vi "Periodic Tasks.vi"(8 "error in":errorcluster) -> ()   [LabVIEW 2019]
doc: "This VI runs in parallel to other tasks. It can contain as many user-defined periodic loops as you need. These can carry out PID or other sorts of timed response."
uses:
  <vilib>/Rock Robotics/WPI/Utilities/WPI_GetSetVariantRefNum.vi
  Robot Global Data.vi
  <vilib>/Rock Robotics/Network Tables/NT Read Number.vi
  <vilib>/Rock Robotics/Network Tables/NT Write Number.vi
  <vilib>/Rock Robotics/WPI/Ultrasonic/WPI_SonarSRF04DigitalGetRange.vi
  <vilib>/Rock Robotics/WPI/Ultrasonic/WPI_SonarSRF04DigitalRefNum Registry Get.vi
panel:
  out "Distance":dbl
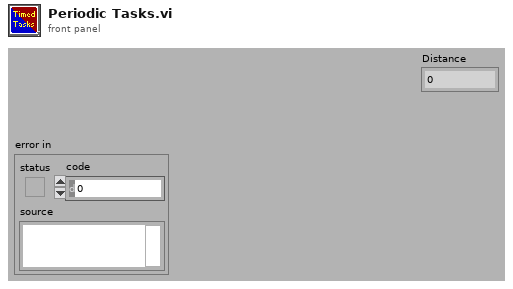
[diagram p1: front panel]
types:
  T1 = typedef "WPI_ServoDeviceRef.ctl" = cluster{"DeviceStatus":errorcluster, "PWM Channel":T2, "DeadBand":T3}
  T2 = typedef "FPGA_DIOPWMChannel.ctl" = enum8{"PWM 0", "PWM 1", "PWM 2", "PWM 3", "PWM 4", "PWM 5", "PWM 6", "PWM 7", "PWM 8", "PWM 9", "PWM MXP 0", "PWM MXP 1", "PWM MXP 2", "PWM MXP 3", "PWM MXP 4", "PWM MXP 5", "PWM MXP 6", "PWM MXP 7", "PWM MXP 8", "PWM MXP 9", "Invalid"}
  T3 = typedef "WPI_PWMDeadband.ctl" = cluster{"Name":string, "maxPositivePwm":i32, "minPositivePwm":i32, "centerPwm":i32, "maxNegativePwm":i32, "minNegativePwm":i32, "angularRange":u16}
  T4 = typedef "WPI_UltrasonicDeviceRef.ctl" = cluster{"DevStatus":errorcluster, "Ping Channel":T5, "Echo Channel":T5, "CntIndex":T6}
  T5 = typedef "FPGA_DIOChannel.ctl" = enum8{"DIO 0", "DIO 1", "DIO 2", "DIO 3", "DIO 4", "DIO 5", "DIO 6", "DIO 7", "DIO 8", "DIO 9", "DIO MXP 0", "DIO MXP 1", "DIO MXP 2", "DIO MXP 3", "DIO MXP 4", "DIO MXP 5", "DIO MXP 6", "DIO MXP 7", "DIO MXP 8", "DIO MXP 9", "DIO MXP 10", "DIO MXP 11", "DIO MXP 12", "DIO MXP 13", "DIO MXP 14", "DIO MXP 15", "SPI Port CS1", "SPI Port CS2", "SPI Port CS3", "SPI Port MISO", "SPI Port MOSI", "Invalid"}
  T6 = typedef "FPGA_CounterCtrSystemIndex.ctl" = enum8{"Ctr 0", "Ctr 1", "Ctr 2", "Ctr 3", "Ctr 4", "Ctr 5", "Ctr 6", "Ctr 7", "Invalid"}
  T7 = typedef "WPI_JoystickDevRef.ctl" = cluster{"Device":T8}
  T8 = typedef "WPI_JoystickDeviceEnum.ctl" = enum16{"USB 0", "USB 1", "USB 2", "USB 3", "USB 4", "USB 5"}
  T9 = typedef "WPI_RobotDriveDevRef.ctl" = cluster{"DevStatus":errorcluster, "Motors[]":T10[], "Square Inputs":bool, "Max Output":dbl}
  T10 = typedef "WPI_MotorControlDeviceRef.ctl" = cluster{"DeviceStatus":errorcluster, "Type":T11, "PWM":cluster{"PWM Channel":T2, "DeadBand":T3}, "CAN":cluster{"Device Number":u8, "SetOutput VI Ref":variant, "GetOutput VI Ref":variant, "Enable VI Ref":variant, "Disable VI Ref":variant, "Data":variant}, "Invert":bool, "DIO PWM":cluster{"PWM \"Enable\" Channel":T2, "DIOChannel":T5, "PWM Rate":dbl}}
  T11 = typedef "WPI_MotorControlType.ctl" = enum16{"PWM", "CAN", "DIO PWM"}
  T12 = typedef "WPI_GyroDevRef.ctl" = cluster{"DevStatus":errorcluster, "Analog Channel":T13, "Gain (VoltsPerDegree/Second)":dbl, "Gyro Type":enum16{"Analog", "XRS450"}, "Handle":i32, "SPI Bus":T14, "Device Found":bool, "Sample Rate":dbl, "Calibrate On Open":bool, "Offset":dbl}
  T13 = typedef "FPGA_AIChannel.ctl" = enum8{"AI 0", "AI 1", "AI 2", "AI 3", "AI MXP 0", "AI MXP 1", "AI MXP 2", "AI MXP 3", "Invalid"}
  T14 = typedef "spi_bus.ctl" = enum16{"SPI On-Board, CS0", "SPI On-Board, CS1", "SPI On-Board, CS2", "SPI On-Board, CS3", "SPI MXP", "Invalid"}
  T15 = cluster{"JoystickDevRef":T7, "RobotDriveDevRef":T9}
  T16 = typedef "WPI_EncoderDevRef.ctl" = cluster{"DevStatus":errorcluster, "EncoderIndex":T17, "CounterIndex":T6, "DistancePerCount":dbl, "Decoding Type":T18}
  T17 = typedef "FPGA_EncoderIdx.ctl" = enum8{"Enc 0", "Enc 1", "Enc 2", "Enc 3", "Enc 4", "Enc 5", "Enc 6", "Enc 7", "Invalid"}
  T18 = typedef "WPI_EncoderType.ctl" = enum16{"1x", "2x", "4x"}
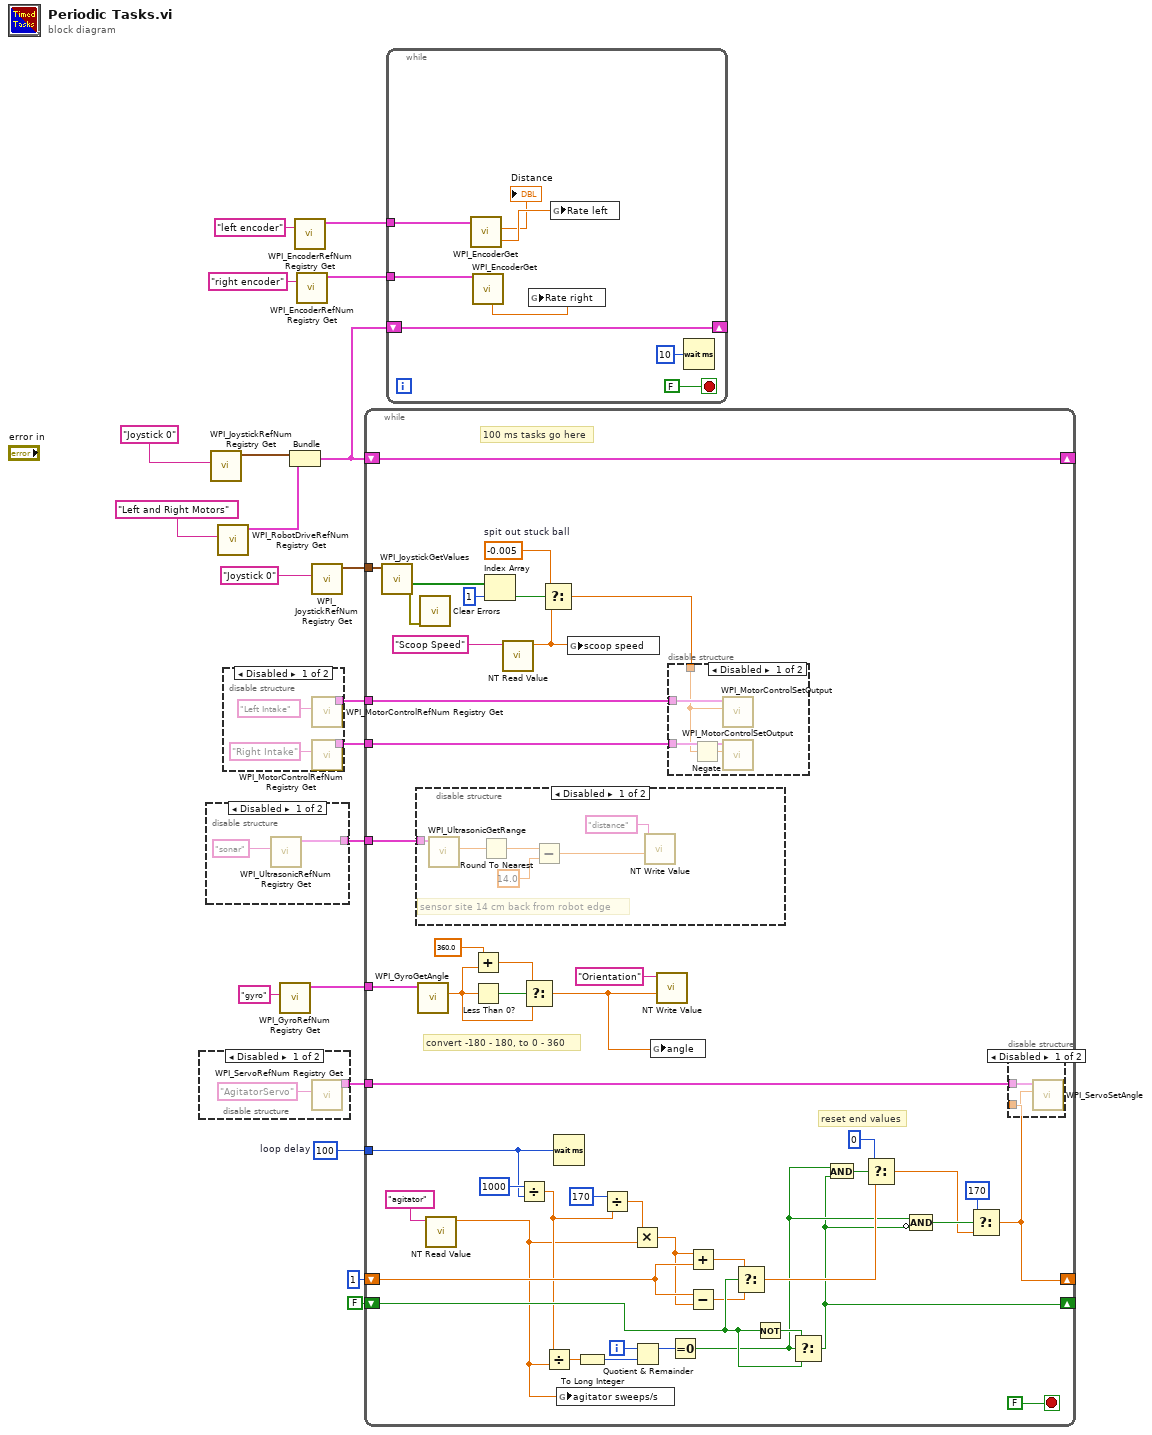
[diagram p0: block diagram]
diagram:
  w8 = u32 100  # loop delay
  n1 = disable-structure shown="Disabled" {
    disable-tunnel: [w21 _] -> w15
    frame Disabled {
      n2 = call <vilib>:"WPI_ServoRefNum Registry Get.vi"("refnum name"="AgitatorServo") -> ("ServoDeviceRef"=w21:T1)  [unwired: 9 in, 1 out]
    }
    frame Enabled {
    }
  }
  n3 = disable-structure shown="Disabled" {
    disable-tunnel: [w23 _] -> w7
    frame Disabled {
      n4 = call-poly <vilib>:"WPI_UltrasonicRefNum Registry Get.vi"("refnum name"="sonar") -> ("SonarSRF04DevRef"=w23:T4)  [unwired: 9 in, 1 out]
    }
    frame Enabled {
    }
  }
  n5 = call <vilib>:"WPI_JoystickRefNum Registry Get.vi"("refnum name"="Joystick 0") -> ("JoystickDevRef"=w18:T7)  [unwired: 1 in, 9 out]
  n6 = call <vilib>:"WPI_RobotDriveRefNum Registry Get.vi"("refnum name"="Left and Right Motors") -> ("RobotDriveDevRef"=w17:T9)  [unwired: 1 in, 9 out]
  n7 = disable-structure shown="Disabled" {
    disable-tunnel: [w28 _] -> w12
    disable-tunnel: [w25 _] -> w11
    frame Disabled {
      n8 = call <vilib>:"WPI_MotorControlRefNum Registry Get.vi"("refnum name"="Left Intake") -> ("MotorControlDevRef"=w28:T10)  [unwired: 9 in, 1 out]
      n9 = call <vilib>:"WPI_MotorControlRefNum Registry Get.vi"("refnum name"="Right Intake") -> ("MotorControlDevRef"=w25:T10)  [unwired: 9 in, 1 out]
    }
    frame Enabled {
    }
  }
  n10 = call <vilib>:"WPI_GyroRefNum Registry Get.vi"("refnum name"="gyro") -> ("GyroDevRef"=w5:T12)  [unwired: 9 in, 1 out]
  n11 = Bundle("JoystickDevRef"=w18, "RobotDriveDevRef"=w17) -> (w16:T15)  [unwired: 1 out]
  n12 = call <vilib>:"WPI_EncoderRefNum Registry Get.vi"("refnum name"="left encoder") -> ("EncoderDevRef"=w1:T16)  [unwired: 9 in, 1 out]
  n13 = call <vilib>:"WPI_EncoderRefNum Registry Get.vi"("refnum name"="right encoder") -> ("EncoderDevRef"=w4:T16)  [unwired: 9 in, 1 out]
  n14 = call <vilib>:"WPI_JoystickRefNum Registry Get.vi"("refnum name"="Joystick 0") -> ("JoystickDevRef"=w9:T7)  [unwired: 1 in, 9 out]
  n15 = while {
    shift-right: [w75] -> _
    shift-left: w16 -> [w75]
    tunnel: w15 -> [w74]
    shift-right: [w43] -> _
    shift-left: 1 ("Angle") -> [w57]
    shift-right: [w46] -> _
    shift-left: FALSE -> [w62]
    tunnel: w12 -> [w70]
    tunnel: w11 -> [w69]
    tunnel: w9 -> [w68]
    tunnel: w8 -> [w59]
    tunnel: w7 -> [w39]
    tunnel: w5 -> [w38]
    i -> [w73]
    stop <- FALSE stop-if-true
    w63 = -0.005  # spit out stuck ball
    # "convert -180 - 180, to 0 - 360"
    # "reset end values"
    # "100 ms tasks go here"
    n16 = call <vilib>:"WPI_JoystickGetValues.vi"("JoystickDevRef"=w68) -> ("error out"=w30:errorcluster, "Buttons"=w67:bool[])  [unwired: 6 in, 3 out]
    n17 = disable-structure shown="Disabled" {
      disable-tunnel: w39 -> [w88 _]
      frame Disabled {
        # "sensor site 14 cm back from robot edge"
        n18 = call-poly <vilib>:"WPI_UltrasonicGetRange.vi"("UltrasonicDevRef"=w88) -> ("Distance"=w87:dbl)  [unwired: 8 in, 2 out]
        n19 = Round To Nearest(number=w87) -> (nearest integer value=w85:dbl)
        n20 = Subtract(x=w85, y=14.0) -> (x-y=w84:dbl)
        n21 = call-poly <vilib>:"NT Write Value.vi"("Numeric"=w84, "Name"="distance") -> ()  [unwired: 9 in, 1 out]
      }
      frame Enabled {
      }
    }
    n22 = call <vilib>:"WPI_GyroGetAngle.vi"("GyroDevRef"=w38) -> ("Angle"=w34:dbl)  [unwired: 6 in, 4 out]
    n23 = call <vilib>:"Clear Errors.vi"("error in (no error)"=w30) -> ()  [unwired: 5 in, 2 out]
    n24 = call-poly <vilib>:"NT Read Value.vi"("Name"="agitator") -> ("Numeric"=w31:dbl)  [unwired: 9 in, 1 out]
    n25 = Add(x=360.0, y=w34) -> (x+y=w35:dbl)
    n26 = Less Than 0?(x=w34) -> (x < 0?=w36:bool)
    n27 = Index Array(array=w67, index=1) -> (element=w65:bool)
    n28 = call-poly <vilib>:"NT Read Value.vi"("Name"="Scoop Speed") -> ("Numeric"=w40:dbl)  [unwired: 9 in, 1 out]
    n29 = Divide(x=u32 1000 ("loop delay"), y=w59) -> (x/y=w55:dbl)
    n30 = Select(t=w35, s=w36, f=w34) -> (s? t:f=w29:dbl)
    n31 = Select(t=w63, s=w65, f=w40) -> (s? t:f=w64:dbl)
    n32 = Divide(x=w55, y=w31) -> (x/y=w53:dbl)
    n33 = Wait (ms)(milliseconds to wait=w59) -> ()  [unwired: 1 out]
    n34 = global write "Robot Global Data.vi" "agitator sweeps/s"(w31) -> ()
    n35 = global write "Robot Global Data.vi" "scoop speed"(w40) -> ()
    n36 = To Long Integer(number=w53) -> (32bit integer=w51:i32)
    n37 = Divide(x=170 ("y"), y=w55) -> (x/y=w54:dbl)
    n38 = Multiply(x=w54, y=w31) -> (x*y=w52:dbl)
    n39 = Quotient & Remainder(x=w73, y=w51) -> (x-y*floor(x/y)=w72:i32)  [unwired: 1 out]
    n40 = global write "Robot Global Data.vi" "angle"(w29) -> ()
    n41 = call-poly <vilib>:"NT Write Value.vi"("Numeric"=w29, "Name"="Orientation") -> ()  [unwired: 9 in, 1 out]
    n42 = disable-structure shown="Disabled" {
      disable-tunnel: w70 -> [w82 _]
      disable-tunnel: w69 -> [w81 _]
      disable-tunnel: w64 -> [w79 _]
      frame Disabled {
        n43 = Negate(x=w79) -> (-x=w80:dbl)
        n44 = call <vilib>:"WPI_MotorControlSetOutput.vi"("Output"=w79, "MotorControlDevRef"=w82) -> ()  [unwired: 7 in, 3 out]
        n45 = call <vilib>:"WPI_MotorControlSetOutput.vi"("Output"=w80, "MotorControlDevRef"=w81) -> ()  [unwired: 7 in, 3 out]
      }
      frame Enabled {
      }
    }
    n46 = Equal To 0?(x=w72) -> (x = 0?=w47:bool)
    n47 = Add(x=w52, y=w57) -> (x+y=w58:dbl)
    n48 = Subtract(x=w57, y=w52) -> (x-y=w61:dbl)
    n49 = Select(t=w58, s=w62, f=w61) -> (s? t:f=w48:dbl)
    n50 = Not(x=w62) -> (.not. x?=w71:bool)
    n51 = Select(t=w71, s=w47, f=w62) -> (s? t:f=w46:bool)
    n52 = And(x=w47, y=w46) -> (x .and. y?=w50:bool)
    n53 = Select(t=0 ("y"), s=w50, f=w48) -> (s? t:f=w44:dbl)
    n54 = Compound Arithmetic op=AND(w47, invert w46) -> (w45:bool)
    n55 = Select(t=170 ("y"), s=w45, f=w44) -> (s? t:f=w43:dbl)
    n56 = disable-structure shown="Disabled" {
      disable-tunnel: w74 -> [w78 _]
      disable-tunnel: w43 -> [w77 _]
      frame Disabled {
        n57 = call <vilib>:"WPI_ServoSetAngle.vi"("Angle"=w77, "ServoDeviceRef"=w78) -> ()  [unwired: 8 in, 2 out]
      }
      frame Enabled {
      }
    }
  }
  n58 = while {
    shift-right: [w93] -> _
    shift-left: w16 -> [w93]
    tunnel: w4 -> [w94]
    tunnel: w1 -> [w91]
    stop <- FALSE stop-if-true
    n59 = call <vilib>:"WPI_EncoderGet.vi"("EncoderDevRef"=w91) -> ("Distance"=→"Distance":dbl, "Rate"=w90:dbl)  [unwired: 5 in, 4 out]
    n60 = call <vilib>:"WPI_EncoderGet.vi"("EncoderDevRef"=w94) -> ("Rate"=w92:dbl)  [unwired: 5 in, 5 out]
    n61 = global write "Robot Global Data.vi" "Rate right"(w92) -> ()
    n62 = global write "Robot Global Data.vi" "Rate left"(w90) -> ()
    n63 = Wait (ms)(milliseconds to wait=u32 10) -> ()  [unwired: 1 out]
  }
